vi "ApplyInstrument_v2.vi"(0 "Instrument":string, 1 "ITC ref":T1={"ITC"=0, "Signal"=enum."Sensor 3"}, 2 "Conversion Factor Fix\n1 V = ??":dbl=1.0, 3 "K2400 1":refnum<visa-resource-name>, 4 "Sweep Instrument":string(combo), 5 "Valin":dbl, 6 "Fix Instrument":string(combo), 7 "DAC COM port":refnum<visa-resource-name>="COM1", 8 "VI4 Instrument":string(combo), 9 "IOL Instrument":string(combo), 11 "error in (no error)":errorcluster, 12 "K2400 2":refnum<visa-resource-name>, 13 "Conversion Factor Sweep\n1 V = ??":dbl=1.0, 14 "Lockin1":refnum<visa-resource-name>="GPIB0::7") -> (15 "error out":errorcluster)   [LabVIEW 2011]
uses:
  Kelvinox drivers/ITCAPPS - Copie.LLB/ITCSignal.ctl
  Kelvinox drivers/ITCAPPS.LLB/ITCSignals.ctl
  GlobalVar.vi
  monochromatorcontrol/perHandlemonochromator.vi
  monochromatorcontrol/libPhyspec.lvlib
panel:
  out "concatenated string 2":string
  out "concatenated string":string
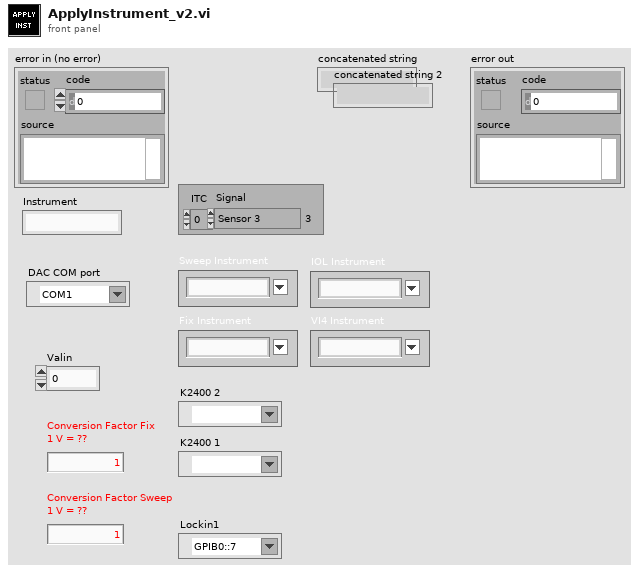
[diagram p1: front panel]
types:
  T1 = typedef "ITCSignal.ctl" = cluster{"ITC":u16, "Signal":T2}
  T2 = typedef "ITCSignals.ctl" = enum16{"Setpoint", "Sensor 1", "Sensor 2", "Sensor 3", "Needle Valve %", "Heater %"}
  T3 = cluster{"Power Stabilization":bool, "Laser Power [W]":dbl, "Power precision":dbl}
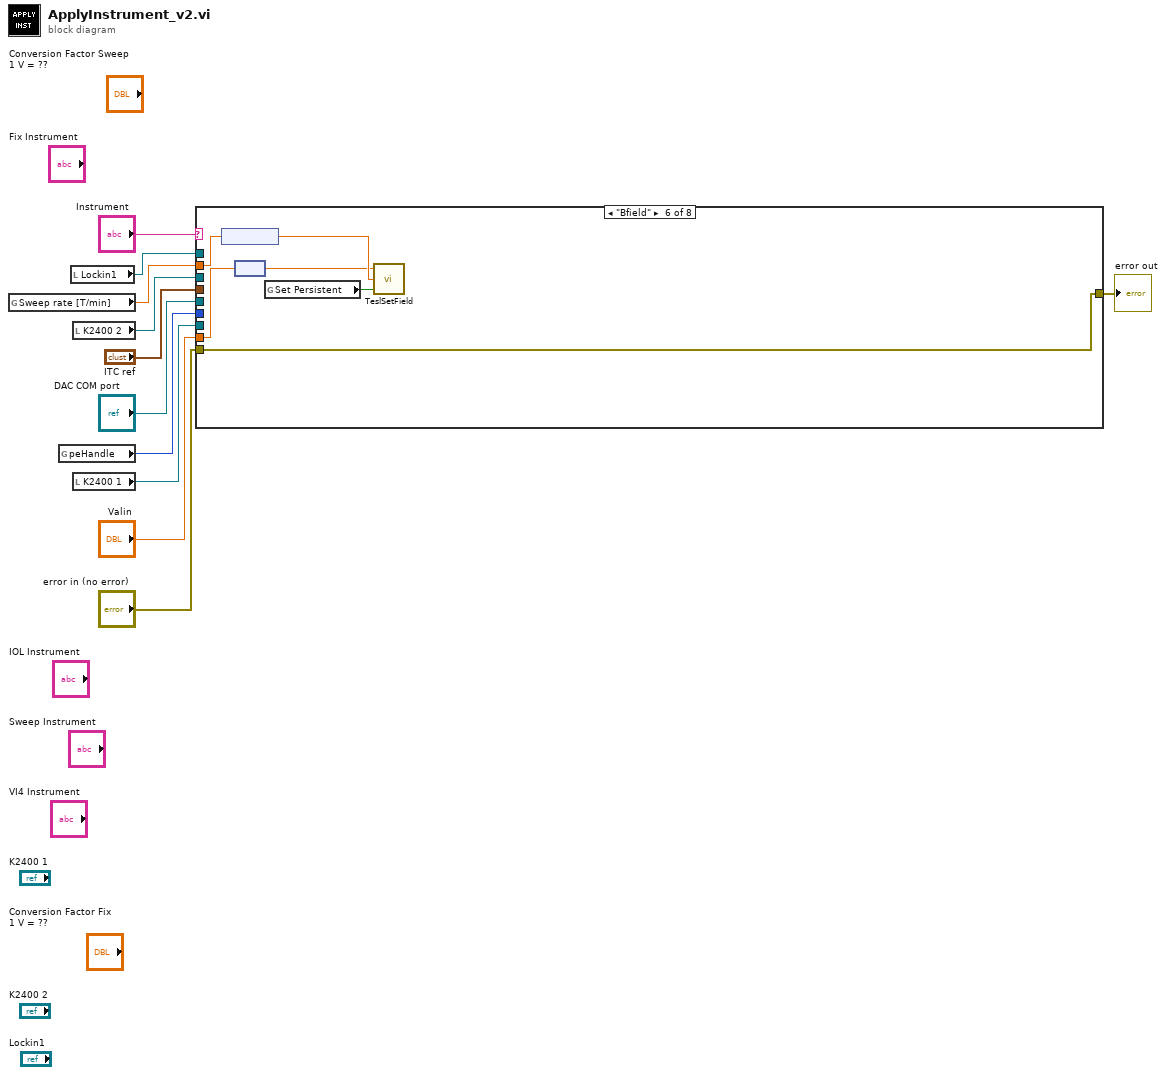
[diagram p0: block diagram]
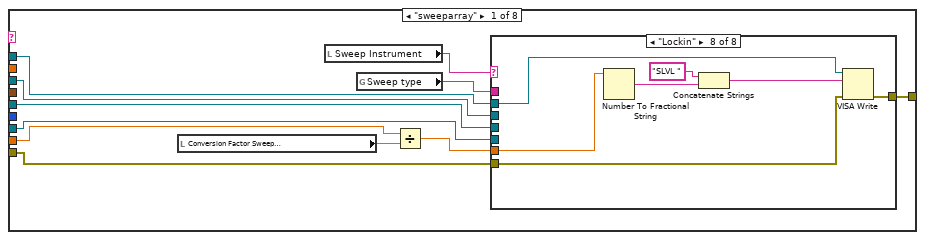
[diagram p2: hidden frame]
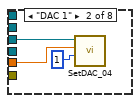
[diagram p4: hidden frame]
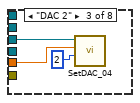
[diagram p5: hidden frame]
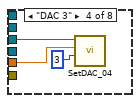
[diagram p6: hidden frame]
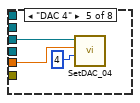
[diagram p7: hidden frame]
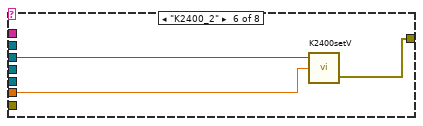
[diagram p8: hidden frame]
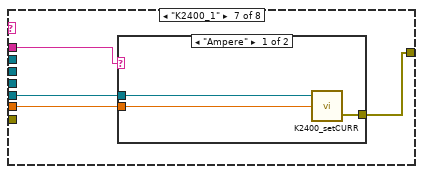
[diagram p9: hidden frame]
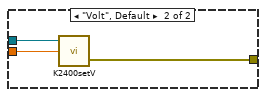
[diagram p10: hidden frame]
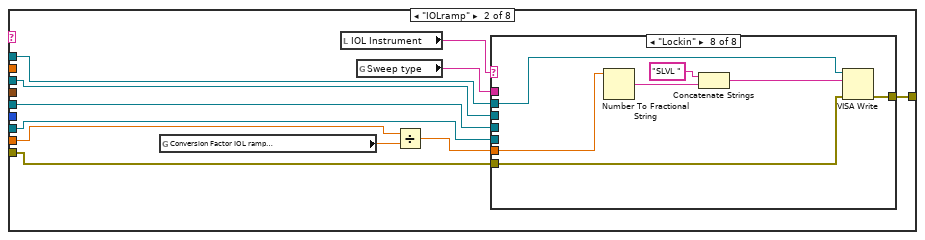
[diagram p11: hidden frame]
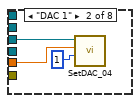
[diagram p13: hidden frame]
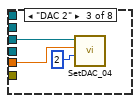
[diagram p14: hidden frame]
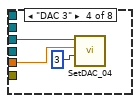
[diagram p15: hidden frame]
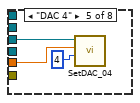
[diagram p16: hidden frame]
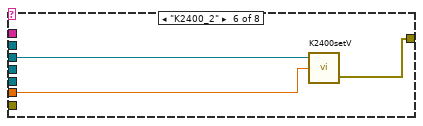
[diagram p17: hidden frame]
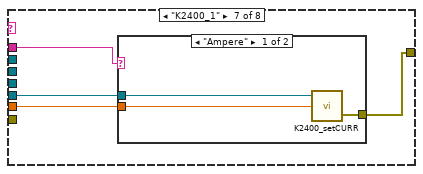
[diagram p18: hidden frame]
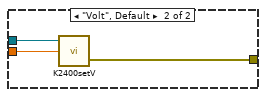
[diagram p19: hidden frame]
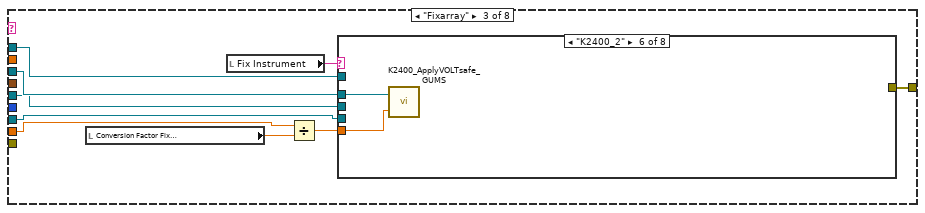
[diagram p20: hidden frame]
diagram:
  n1 = global read "GlobalVar.vi" "Sweep rate [T/min]"() -> (w2:dbl)
  n2 = global read "perHandlemonochromator.vi" "peHandle"() -> (w1:u32)
  n3 = local read "Lockin1"() -> (w11:refnum<visa-resource-name>)
  n4 = local read "K2400 2"() -> (w10:refnum<visa-resource-name>)
  n5 = local read "K2400 1"() -> (w9:refnum<visa-resource-name>)
  n6 = case shown="\"Bfield\"" "Instrument" {
    tunnel: "Valin" -> [w22 w65 w106 w137 _ w166 w177 w190]
    tunnel: "ITC ref" -> [_ _ _ _ _ _ w176 _]
    tunnel: w11 -> [w20 w63 w104 w135 _ _ _ _]
    tunnel: w10 -> [w19 w62 w103 w134 _ _ _ _]
    tunnel: w9 -> [w18 w61 w102 w133 _ _ _ _]
    tunnel: w2 -> [_ _ _ _ _ w164 _ _]
    tunnel: "error in (no error)" -> [w16 w59 _ _ w160 w163 w170 w199]
    tunnel: [w15 w58 w100 w131 w160 w163 w171 w196] -> w4
    tunnel: "DAC COM port" -> [w14 w57 w99 w130 _ _ _ _]
    tunnel: w1 -> [_ _ _ _ _ _ _ w200]
    frame "sweeparray" {
      n7 = local read "Conversion Factor Sweep\n1 V = ??"() -> (w12:dbl)
      n8 = local read "Sweep Instrument"() -> (w17:string)
      n9 = global read "GlobalVar.vi" "Sweep type"() -> (w13:string)
      n10 = Divide(x=w22, y=w12) -> (x/y=w21:dbl)
      n11 = case shown="\"Lockin\"" w17 {
        tunnel: w21 -> [_ w25 w28 w31 w34 w37 w41 w51]
        tunnel: [_ _ _ _ _ w35 w40 w50] -> w15
        tunnel: w20 -> [_ _ _ _ _ _ _ w49]
        tunnel: w19 -> [_ _ _ _ _ w36 _ _]
        tunnel: w18 -> [_ _ _ _ _ _ w39 _]
        tunnel: w16 -> [_ _ _ _ _ _ _ w48]
        tunnel: w14 -> [_ w23 w26 w29 w32 _ _ _]
        tunnel: w13 -> [_ _ _ _ _ _ w38 _]
        frame Default {
        }
        frame "DAC 1" {
          n12 = call "SetDAC_04.vi"("RS232/ Optical Fiber"=w23, "DATA (V)"=w25, "DAC nr"=u8 1) -> ()  [unwired: 2 in, 1 out]
        }
        frame "DAC 2" {
          n13 = call "SetDAC_04.vi"("RS232/ Optical Fiber"=w26, "DATA (V)"=w28, "DAC nr"=u8 2) -> ()  [unwired: 2 in, 1 out]
        }
        frame "DAC 3" {
          n14 = call "SetDAC_04.vi"("RS232/ Optical Fiber"=w29, "DATA (V)"=w31, "DAC nr"=u8 3) -> ()  [unwired: 2 in, 1 out]
        }
        frame "DAC 4" {
          n15 = call "SetDAC_04.vi"("RS232/ Optical Fiber"=w32, "DATA (V)"=w34, "DAC nr"=u8 4) -> ()  [unwired: 2 in, 1 out]
        }
        frame "K2400_2" {
          n16 = call "K2400setV.vi"("Voltage target [V]"=w37, "VISA Resource Name"=w36) -> ("error out"=w35:errorcluster)  [unwired: 1 in, 1 out]
        }
        frame "K2400_1" {
          n17 = case shown="\"Ampere\"" w38 {
            tunnel: w41 -> [w43 w47]
            tunnel: [w42 w46] -> w40
            tunnel: w39 -> [w44 w45]
            frame "Ampere" {
              n18 = call "K2400_setCURR.vi"("Current [A]"=w43, "GPIB address"=w44) -> ("error out"=w42:errorcluster)  [unwired: 1 in, 1 out]
            }
            frame "Volt", Default {
              n19 = call "K2400setV.vi"("Voltage target [V]"=w47, "VISA Resource Name"=w45) -> ("error out"=w46:errorcluster)  [unwired: 1 in, 1 out]
            }
          }
        }
        frame "Lockin" {
          n20 = Number To Fractional String(number=w51) -> (F-format string=w54:string)  [unwired: 3 out]
          n21 = Concatenate Strings("SLVL " ("chaîne"), w54) -> (w52:string)
          n22 = VISA Write(VISA resource name=w49, write buffer=w52, error in (no error)=w48) -> (error out=w50:errorcluster)  [unwired: 2 out]
        }
      }
    }
    frame "IOLramp" {
      n23 = global read "GlobalVar.vi" "Conversion Factor IOL ramp\n1 V = ??"() -> (w55:dbl)
      n24 = local read "IOL Instrument"() -> (w60:string)
      n25 = global read "GlobalVar.vi" "Sweep type"() -> (w56:string)
      n26 = Divide(x=w65, y=w55) -> (x/y=w64:dbl)
      n27 = case shown="\"Lockin\"" w60 {
        tunnel: w64 -> [_ w68 w71 w74 w77 w80 w84 w94]
        tunnel: [_ _ _ _ _ w78 w83 w93] -> w58
        tunnel: w63 -> [_ _ _ _ _ _ _ w92]
        tunnel: w62 -> [_ _ _ _ _ w79 _ _]
        tunnel: w61 -> [_ _ _ _ _ _ w82 _]
        tunnel: w59 -> [_ _ _ _ _ _ _ w91]
        tunnel: w57 -> [_ w66 w69 w72 w75 _ _ _]
        tunnel: w56 -> [_ _ _ _ _ _ w81 _]
        frame Default {
        }
        frame "DAC 1" {
          n28 = call "SetDAC_04.vi"("RS232/ Optical Fiber"=w66, "DATA (V)"=w68, "DAC nr"=u8 1) -> ()  [unwired: 2 in, 1 out]
        }
        frame "DAC 2" {
          n29 = call "SetDAC_04.vi"("RS232/ Optical Fiber"=w69, "DATA (V)"=w71, "DAC nr"=u8 2) -> ()  [unwired: 2 in, 1 out]
        }
        frame "DAC 3" {
          n30 = call "SetDAC_04.vi"("RS232/ Optical Fiber"=w72, "DATA (V)"=w74, "DAC nr"=u8 3) -> ()  [unwired: 2 in, 1 out]
        }
        frame "DAC 4" {
          n31 = call "SetDAC_04.vi"("RS232/ Optical Fiber"=w75, "DATA (V)"=w77, "DAC nr"=u8 4) -> ()  [unwired: 2 in, 1 out]
        }
        frame "K2400_2" {
          n32 = call "K2400setV.vi"("Voltage target [V]"=w80, "VISA Resource Name"=w79) -> ("error out"=w78:errorcluster)  [unwired: 1 in, 1 out]
        }
        frame "K2400_1" {
          n33 = case shown="\"Ampere\"" w81 {
            tunnel: w84 -> [w86 w90]
            tunnel: [w85 w89] -> w83
            tunnel: w82 -> [w87 w88]
            frame "Ampere" {
              n34 = call "K2400_setCURR.vi"("Current [A]"=w86, "GPIB address"=w87) -> ("error out"=w85:errorcluster)  [unwired: 1 in, 1 out]
            }
            frame "Volt", Default {
              n35 = call "K2400setV.vi"("Voltage target [V]"=w90, "VISA Resource Name"=w88) -> ("error out"=w89:errorcluster)  [unwired: 1 in, 1 out]
            }
          }
        }
        frame "Lockin" {
          n36 = Number To Fractional String(number=w94) -> (F-format string=w97:string)  [unwired: 3 out]
          n37 = Concatenate Strings("SLVL " ("chaîne"), w97) -> (w95:string)
          n38 = VISA Write(VISA resource name=w92, write buffer=w95, error in (no error)=w91) -> (error out=w93:errorcluster)  [unwired: 2 out]
        }
      }
    }
    frame "Fixarray" {
      n39 = local read "Conversion Factor Fix\n1 V = ??"() -> (w98:dbl)
      n40 = local read "Fix Instrument"() -> (w101:string)
      n41 = Divide(x=w106, y=w98) -> (x/y=w105:dbl)
      n42 = case shown="\"K2400_2\"" w101 {
        tunnel: w105 -> [_ w108 w111 w114 w117 w119 w121 w125]
        tunnel: [_ _ _ _ _ _ _ w124] -> w100
        tunnel: w104 -> [_ _ _ _ _ _ _ w123]
        tunnel: w103 -> [_ _ _ _ _ w120 _ _]
        tunnel: w102 -> [_ _ _ _ _ _ w122 _]
        tunnel: w99 -> [_ w109 w112 w115 w118 _ _ _]
        frame Default {
        }
        frame "DAC 1" {
          n43 = call "SetDAC_04.vi"("RS232/ Optical Fiber"=w109, "DATA (V)"=w108, "DAC nr"=u8 1) -> ()  [unwired: 2 in, 1 out]
        }
        frame "DAC 2" {
          n44 = call "SetDAC_04.vi"("RS232/ Optical Fiber"=w112, "DATA (V)"=w111, "DAC nr"=u8 2) -> ()  [unwired: 2 in, 1 out]
        }
        frame "DAC 3" {
          n45 = call "SetDAC_04.vi"("RS232/ Optical Fiber"=w115, "DATA (V)"=w114, "DAC nr"=u8 3) -> ()  [unwired: 2 in, 1 out]
        }
        frame "DAC 4" {
          n46 = call "SetDAC_04.vi"("RS232/ Optical Fiber"=w118, "DATA (V)"=w117, "DAC nr"=u8 4) -> ()  [unwired: 2 in, 1 out]
        }
        frame "K2400_2" {
          n47 = call "K2400_ApplyVOLTsafe_GUMS.vi"("Voltage target [V]"=w119, "VISA Resource Name"=w120) -> ()  [unwired: 1 in]
        }
        frame "K2400_1" {
          n48 = call "K2400_ApplyVOLTsafe_GUMS.vi"("Voltage target [V]"=w121, "VISA Resource Name"=w122) -> ()  [unwired: 1 in]
        }
        frame "Lockin" {
          n49 = Number To Fractional String(number=w125) -> (F-format string=w128:string)  [unwired: 3 out]
          n50 = Concatenate Strings("SLVL " ("chaîne"), w128) -> (w126:string)
          "concatenated string" <- w126
          n51 = VISA Write(VISA resource name=w123, write buffer=w126) -> (error out=w124:errorcluster)  [unwired: 1 in, 2 out]
        }
      }
    }
    frame "VI4array" {
      n52 = global read "GlobalVar.vi" "Conversion Factor VI 4\n1 V = ??"() -> (w129:dbl)
      n53 = local read "VI4 Instrument"() -> (w132:string)
      n54 = Divide(x=w137, y=w129) -> (x/y=w136:dbl)
      n55 = case shown="\"DAC 3\"" w132 {
        tunnel: w136 -> [_ w139 w142 w145 w148 w150 w152 w156]
        tunnel: [_ _ _ _ _ _ _ w155] -> w131
        tunnel: w135 -> [_ _ _ _ _ _ _ w154]
        tunnel: w134 -> [_ _ _ _ _ w151 _ _]
        tunnel: w133 -> [_ _ _ _ _ _ w153 _]
        tunnel: w130 -> [_ w140 w143 w146 w149 _ _ _]
        frame Default {
        }
        frame "DAC 1" {
          n56 = call "SetDAC_04.vi"("RS232/ Optical Fiber"=w140, "DATA (V)"=w139, "DAC nr"=u8 1) -> ()  [unwired: 2 in, 1 out]
        }
        frame "DAC 2" {
          n57 = call "SetDAC_04.vi"("RS232/ Optical Fiber"=w143, "DATA (V)"=w142, "DAC nr"=u8 2) -> ()  [unwired: 2 in, 1 out]
        }
        frame "DAC 3" {
          n58 = call "SetDAC_04.vi"("RS232/ Optical Fiber"=w146, "DATA (V)"=w145, "DAC nr"=u8 3) -> ()  [unwired: 2 in, 1 out]
        }
        frame "DAC 4" {
          n59 = call "SetDAC_04.vi"("RS232/ Optical Fiber"=w149, "DATA (V)"=w148, "DAC nr"=u8 4) -> ()  [unwired: 2 in, 1 out]
        }
        frame "K2400_2" {
          n60 = call "K2400_ApplyVOLTsafe_GUMS.vi"("Voltage target [V]"=w150, "VISA Resource Name"=w151) -> ()  [unwired: 1 in]
        }
        frame "K2400_1" {
          n61 = call "K2400_ApplyVOLTsafe_GUMS.vi"("Voltage target [V]"=w152, "VISA Resource Name"=w153) -> ()  [unwired: 1 in]
        }
        frame "Lockin" {
          n62 = Number To Fractional String(number=w156) -> (F-format string=w159:string)  [unwired: 3 out]
          n63 = Concatenate Strings("SLVL " ("chaîne"), w159) -> (w157:string)
          "concatenated string 2" <- w157
          n64 = VISA Write(VISA resource name=w154, write buffer=w157) -> (error out=w155:errorcluster)  [unwired: 1 in, 2 out]
        }
      }
    }
    frame Default {
      n65 = Wait (ms)(milliseconds to wait=u32 2000) -> ()  [unwired: 1 out]
    }
    frame "Bfield" {
      n66 = node(w164) -> (w167:dbl[unit])
      n67 = node(w166) -> (w165:dbl[unit])
      n68 = global read "GlobalVar.vi" "Set Persistent"() -> (w162:bool)
      n69 = call "TeslSetField.vi"("Set Persistent"=w162, "Sweep rate"=w167, "Field required:"=w165) -> ()  [unwired: 1 in, 2 out]
    }
    frame "Temperature" {
      n70 = global read "GlobalVar.vi" "T rate [K/min]"() -> (w168:dbl)
      n71 = Equal To 0?(x=w168) -> (x = 0?=w169:bool)
      n72 = case shown="False" w169 {
        tunnel: w177 -> [w180 w186]
        tunnel: w176 -> [w181 w184]
        tunnel: [w179 w183] -> w175
        tunnel: w168 -> [w178 _]
        frame False {
          n73 = call "ITCGetReading.vi"("Signal"=w181) -> ("Reading"=w182:dbl)  [unwired: 6 in]
          n74 = call "Trampsimple.vi"("Rate [K/min]"=w178, "T stop [K]"=w180, "T start [K]"=w182, "ITCSignal"=w181) -> ("Finished"=w179:bool)  [unwired: 6 in, 1 out]
        }
        frame True {
          n75 = call "Tloop.vi"("ITCSignal"=w184, "T target [K]"=w186, "Regulate ?"=TRUE) -> ("Finish"=w183:bool)  [unwired: 2 in, 1 out]
        }
      }
      n76 = global read "GlobalVar.vi" "Stabilization Time (s)"() -> (w174:i32)
      n77 = Multiply(x=w174, y=1000) -> (x*y=w172:i32)
      n78 = case shown="True" w175 {
        tunnel: w172 -> [_ w189]
        tunnel: [w187 w188] -> w171
        tunnel: w170 -> [w187 w188]
        frame False {
        }
        frame True {
          n79 = Wait (ms)(milliseconds to wait=w189) -> ()  [unwired: 1 out]
        }
      }
    }
    frame "wavelength" {
      n80 = call "PE Set Wavelength.vi"("error in (no error)"=w199, "wavelength"=w190, "peHandle"=w200) -> ("error out"=w192:errorcluster)  [unwired: 7 in, 1 out]
      n81 = global read "GlobalVar.vi" "PEM present ?"() -> (w193:bool)
      n82 = case shown="True" w193 {
        tunnel: w192 -> [w201 w204]
        tunnel: [w201 w203] -> w191
        tunnel: w190 -> [_ w202]
        frame False {
        }
        frame True {
          n83 = global read "GlobalVar.vi" "PEM VISA"() -> (w205:refnum<visa-resource-name>)
          n84 = call "HindsPEM100_SetWavelength.vi"("VISA refnum in"=w205, "Wavelength (nm)"=w202, "error in (no error)"=w204) -> ("error out"=w203:errorcluster)  [unwired: 15 in, 1 out]
        }
      }
      n85 = global read "GlobalVar.vi" "LaserControl"() -> (w198:T3)
      n86 = Unbundle By Name(w198) -> ("Power Stabilization"=w197:bool, "Laser Power [W]"=w195:dbl, "Power precision"=w194:dbl)
      n87 = case shown="True" w197 {
        tunnel: w191 -> [w206 w210]
        tunnel: [w206 w209] -> w196
        tunnel: w195 -> [_ w208]
        tunnel: w194 -> [_ w207]
        frame False {
        }
        frame True {
          n88 = call "Powerstab.vi"("error out"=w210, "Power precision"=w207, "Laser Power [W]"=w208) -> ("error out 2"=w209:errorcluster)  [unwired: 7 in, 1 out]
        }
      }
    }
  }
  "error out" <- w4
